vi "Save Single turn magnet data.vi"(4 "Save data":bool=TRUE, 6 "Maximum Time (10000ms)":u32=100000, 8 "Error In":errorcluster, 9 "Channel names to save":string[](array[string])=["Bdot", "Signal", "BdotSafe"], 10 "Fetch channels":u16[](array[ring])=[0, 1, 2] items=["Channel 1", "Channel 2", "Channel 3", "Channel 4", "Math", "Reference 1", "Reference 2", "Reference 3", "Reference 4", "D0", "D1", "D2", "D3", "D4", "D5", "D6", "D7", "D8", "D9", "D10", "D11", "D12", "D13", "D14", "D15", "Amplitude", "Frequency", "Phase", "Normal", "Average", "Maximum Peak Hold", "Minimum Peak Hold"], 11 "VISA resource name":refnum<visa-resource-name>="USB0::0x0699::0x0401::C011905::INSTR") -> (0 "Error Out":errorcluster, 2 "Waveform Graph":waveform(dbl)[](graph), 3 "File Path":path)   [LabVIEW 2016]
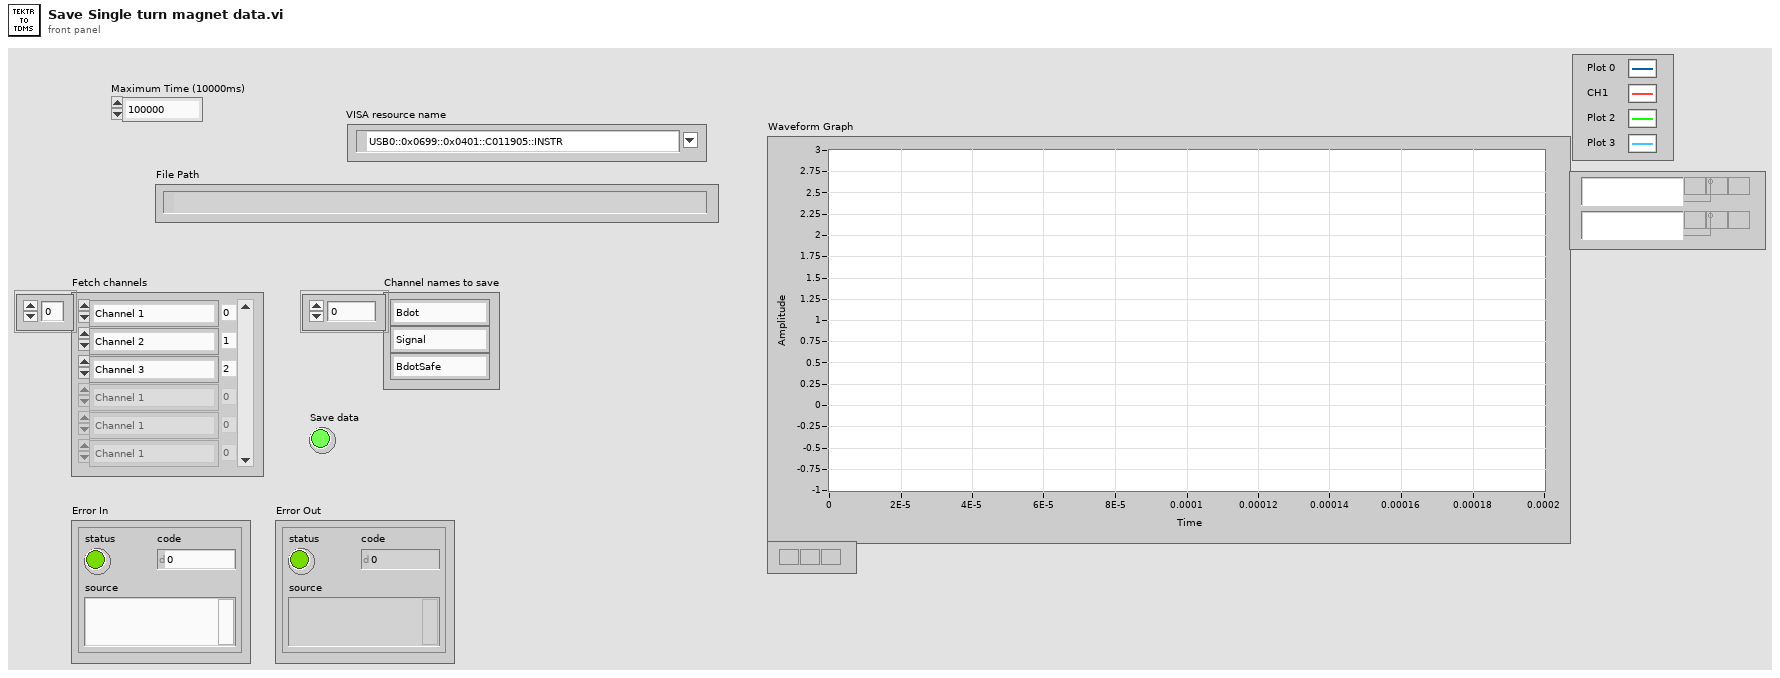
[diagram p1: front panel]
types:
  T1 = enum16{"open", "open or create", "create or replace", "create", "open (read-only)"}
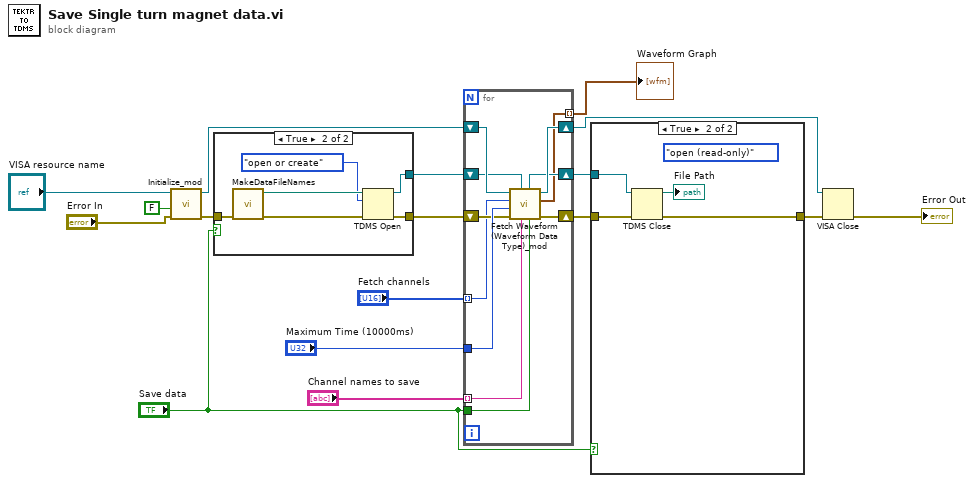
[diagram p0: block diagram]
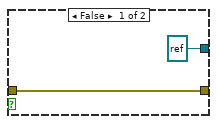
[diagram p3: hidden frame]
diagram:
  n1 = call "Initialize_mod.vi"("error in (no error)"="Error In", "Reset (True)"=FALSE, "VISA resource name"="VISA resource name") -> ("error out"=w12:errorcluster, "VISA resource name out"=w17:refnum<visa-resource-name>)  [unwired: 7 in]
  n2 = case shown="True" "Save data" {
    tunnel: w12 -> [w19 w25]
    tunnel: [w19 w23] -> w11
    tunnel: [refnum<k34> refnum ("tdms file out") w21] -> w10
    frame False {
    }
    frame True {
      n3 = call "MakeDataFileNames.vi"("Error In"=w25) -> ("Error Out"=w24:errorcluster, "Data File  Path"=w22:path)  [unwired: 7 in, 2 out]
      n4 = TDMS Open(8:w24, 10:T1."open or create" ("operation (0:open)"), 11:w22) -> (0:w23:errorcluster, 3:w21:refnum<k34>)  [unwired: 4 in]
    }
  }
  n5 = for {
    tunnel: "Maximum Time (10000ms)" -> [w35]
    tunnel: "Save data" -> [w30]
    tunnel: [w28] -> w3 mode=indexing
    shift-right: [w34] -> w14
    shift-left: w17 -> [w36]
    shift-right: [w31] -> w9
    shift-left: w11 -> [w33]
    shift-right: [w29] -> w6
    shift-left: w10 -> [w32]
    tunnel: "Fetch channels" -> [w27] mode=indexing
    tunnel: "Channel names to save" -> [w26] mode=indexing
    n6 = call "Fetch Waveform (Waveform Data Type)_mod.vi"("Save data"=w30, "Channel name to save"=w26, "tdms file"=w32, "error in (no error)"=w33, "Maximum Time (10000ms)"=w35, "Channel (0: Channel 1)"=w27, "VISA resource name"=w36) -> ("error out"=w31:errorcluster, "Waveform Data"=w28:waveform(dbl), "VISA resource name out"=w34:refnum<visa-resource-name>, "tdms file out"=w29:refnum<k34>)  [unwired: 1 in]
  }
  "Waveform Graph" <- w3
  n7 = case shown="True" "Save data" {
    tunnel: w9 -> [w37 w41]
    tunnel: [w37 w38] -> w8
    tunnel: w6 -> [_ w40]
    frame False {
    }
    frame True {
      (unwired) T1."open (read-only)" ("operation (0:open)")
      n8 = TDMS Close(8:w41, 11:w40) -> (0:w38:errorcluster, 3:→"File Path":path)
    }
  }
  n9 = VISA Close(VISA resource name=w14, error in (no error)=w8) -> (error out=→"Error Out":errorcluster)
